vi "Handle Clocks.vi"(5 "network occupation time":i32=-2, 7 "CLK absolute upper limit":i32=35, 8 "CL2 Clock":i32, 9 "CL1 Clock":i32, 10 "Trigger?":bool=TRUE, 11 "Plant to trigg":enum16{"Plant 1", "Plant 2"}(ring)=enum."Plant 2") -> (0 "CL2 Clock":i32, 1 "CL1 Clock":i32)   [LabVIEW 2016]
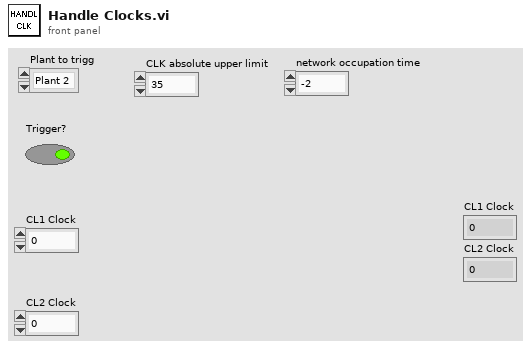
[diagram p1: front panel]
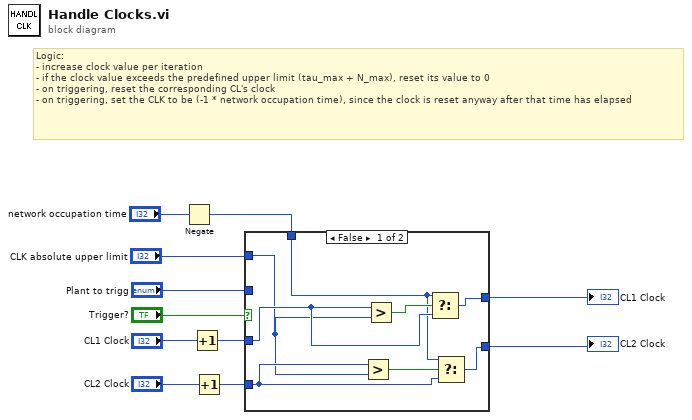
[diagram p0: block diagram]
diagram:
  # "Logic: \n- increase clock value per iteration\n- if the clock value exceeds the predefined upper limit (tau_max + N_max), reset its value to 0\n- on triggering, reset the corresponding CL's clock\n- on triggering, set the CLK to be (-1 * network occupation time), since the clock is reset anyway after that time has elapsed"
  n1 = Negate(x="network occupation time") -> (-x=w1:i32)
  n2 = Increment(x="CL1 Clock") -> (x+1=w7:i32)
  n3 = Increment(x="CL2 Clock") -> (x+1=w6:i32)
  n4 = case shown="False" "Trigger?" {
    tunnel: "Plant to trigg" -> [_ w25]
    tunnel: w7 -> [w18 w23]
    tunnel: w6 -> [w15 w24]
    tunnel: [w14 w21] -> w5
    tunnel: [w17 w22] -> w4
    tunnel: "CLK absolute upper limit" -> [w13 _]
    tunnel: w1 -> [w12 w20]
    frame False {
      n5 = Greater?(x=w15, y=w13) -> (0:w16:bool)
      n6 = Greater?(x=w18, y=w13) -> (0:w19:bool)
      n7 = Select(t=w12, s=w19, f=w18) -> (s? t:f=w17:i32)
      n8 = Select(t=w12, s=w16, f=w15) -> (s? t:f=w14:i32)
    }
    frame True {
      n9 = case shown="\"Plant 1\", Default" w25 {
        tunnel: w24 -> [w26 _]
        tunnel: w23 -> [_ w28]
        tunnel: w20 -> [w27 w29]
        tunnel: [w27 w28] -> w22
        tunnel: [w26 w29] -> w21
        frame "Plant 1", Default {
        }
        frame "Plant 2" {
        }
      }
    }
  }
  "CL1 Clock" <- w4
  "CL2 Clock" <- w5
